vi "CMD_COPY.vi"(6 "Gantry in":refnum<class "Gantry.lvclass">, 8 "error in (no error)":errorcluster, 10 "Arguments":string[](array[string]), 11 "gScript Interpreter in":refnum<class "gScript Interpreter.lvclass">) -> (0 "error out":errorcluster, 3 "gScript Interpreter out":refnum<class "gScript Interpreter.lvclass">, 4 "Gantry out":refnum<class "Gantry.lvclass">)   [LabVIEW 2022 SP3, in "gScript Interpreter.lvclass"]
uses:
  gScript Interpreter.lvclass
  gScript Interpreter.lvclass/gScript Interpreter.ctl
  Shared Components/Gantry Class/Gantry.lvclass
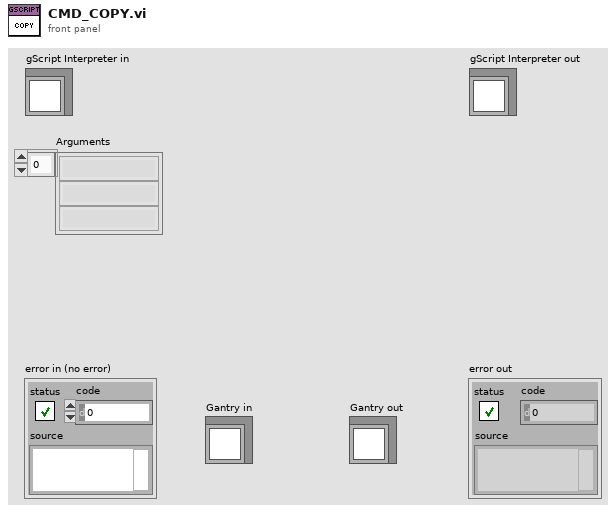
[diagram p1: front panel]
types:
  T1 = typedef "Memory Cell.ctl" = cluster{"type":T2, "x":dbl, "y":dbl, "z":dbl, "w":dbl}
  T2 = typedef "Memory Cell Type Enum.ctl" = enum16{"integer", "float", "vector", "rotation"}
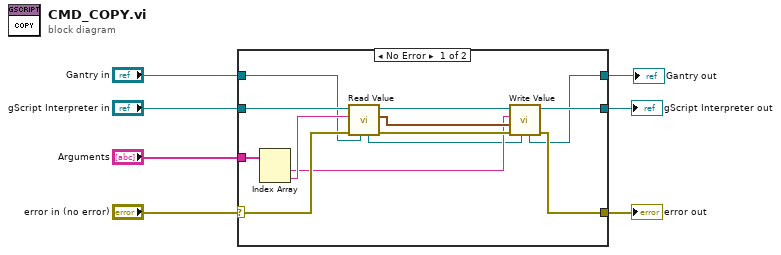
[diagram p0: block diagram]
diagram:
  n1 = case shown="No Error" "error in (no error)" {
    selector: "error in (no error)" -> [w15 w23]
    tunnel: [w13 w23] -> w6
    tunnel: [w16 w22] -> w4
    tunnel: "gScript Interpreter in" -> [w18 w22]
    tunnel: "Arguments" -> [w20 _]
    tunnel: "Gantry in" -> [w10 w21]
    tunnel: [w8 w21] -> w1
    frame No Error {
      n2 = Index Array(array=w20) -> (element #1=w11:string, element #2=w19:string)  [unwired: 2 in]
      n3 = call-dynamic "Read Value.vi"("Gantry in"=w10, "error in (no error)"=w15, "String in"=w19, "gScript Interpreter in"=w18) -> ("error out"=w14:errorcluster, "Memory Cell"=w12:T1, "gScript Interpreter out"=w17:refnum<class "gScript Interpreter.lvclass">, "Gantry out"=w9:refnum<class "Gantry.lvclass">)  [unwired: 4 in]
      n4 = call-dynamic "Write Value.vi"("Gantry in"=w9, "error in (no error)"=w14, "Value"=w12, "Address"=w11, "gScript Interpreter in"=w17) -> ("error out"=w13:errorcluster, "gScript Interpreter out"=w16:refnum<class "gScript Interpreter.lvclass">, "Gantry out"=w8:refnum<class "Gantry.lvclass">)  [unwired: 4 in]
    }
    frame Error {
    }
  }
  "error out" <- w6
  "gScript Interpreter out" <- w4
  "Gantry out" <- w1
